vi "create RT message for sending.vi"(9 "RT data":variant, 10 "RT message":string, 11 "Queues in":T1) -> (3 "Queues out":T1)   [LabVIEW 2018]
uses:
  type defs/Queues.ctl
  supporting VIs/polymorphic VIs/enqueue for comms.vi
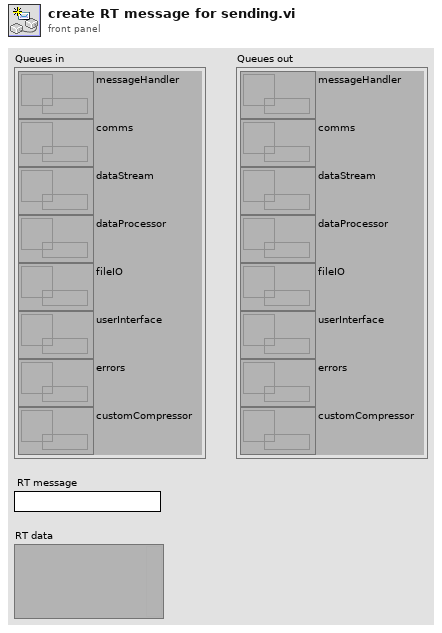
[diagram p1: front panel]
types:
  T1 = typedef "Queues.ctl" = cluster{"messageHandler":refnum<queue>, "comms":refnum<queue>, "dataStream":refnum<queue>, "dataProcessor":refnum<queue>, "fileIO":refnum<queue>, "userInterface":refnum<queue>, "errors":refnum<queue>, "customCompressor":refnum<queue>}
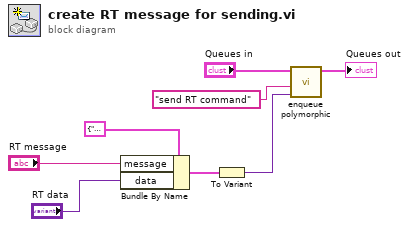
[diagram p0: block diagram]
diagram:
  n1 = Bundle By Name(cluster=cluster{"message":string, "data":variant} {"message"="", "data"=variant}, "message"="RT message", "data"="RT data") -> (w6:cluster{"message":string, "data":variant})
  n2 = To Variant(anything=w6) -> (Variant=w5:variant)
  n3 = call-poly "enqueue polymorphic.vi"("data"=w5, "message"="send RT command", "Queues"="Queues in") -> ("Queues out"=→"Queues out":T1)  [unwired: 8 in]
